vi "RFmx_An_ACP_Disp.vi"(6 "ACP_Values":dbl[](array[numeric]) format="%#_6p", 8 "Int_Bandwidth":dbl[](array[numeric]) format="%#_6p", 9 "Offsets":dbl[](array[numeric]) format="%#_6p", 10 "SignalBandwidth":dbl format="%#_6p", 11 "Input_Waveform":cluster{"x0":dbl, "dx":dbl, "y":sgl[]}) -> (3 "Waveform Graph 2":cluster{"x0":dbl, "dx":dbl, "y":sgl[]}[](graph))   [LabVIEW 2014]
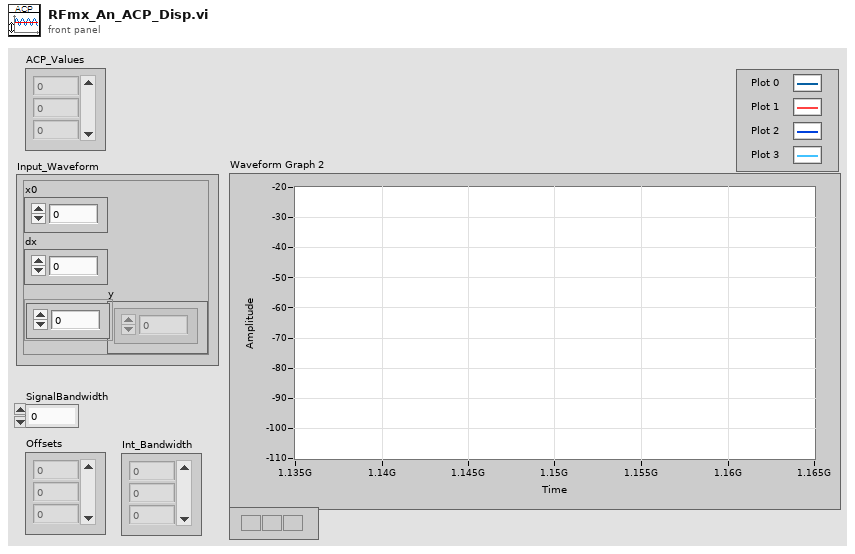
[diagram p1: front panel]
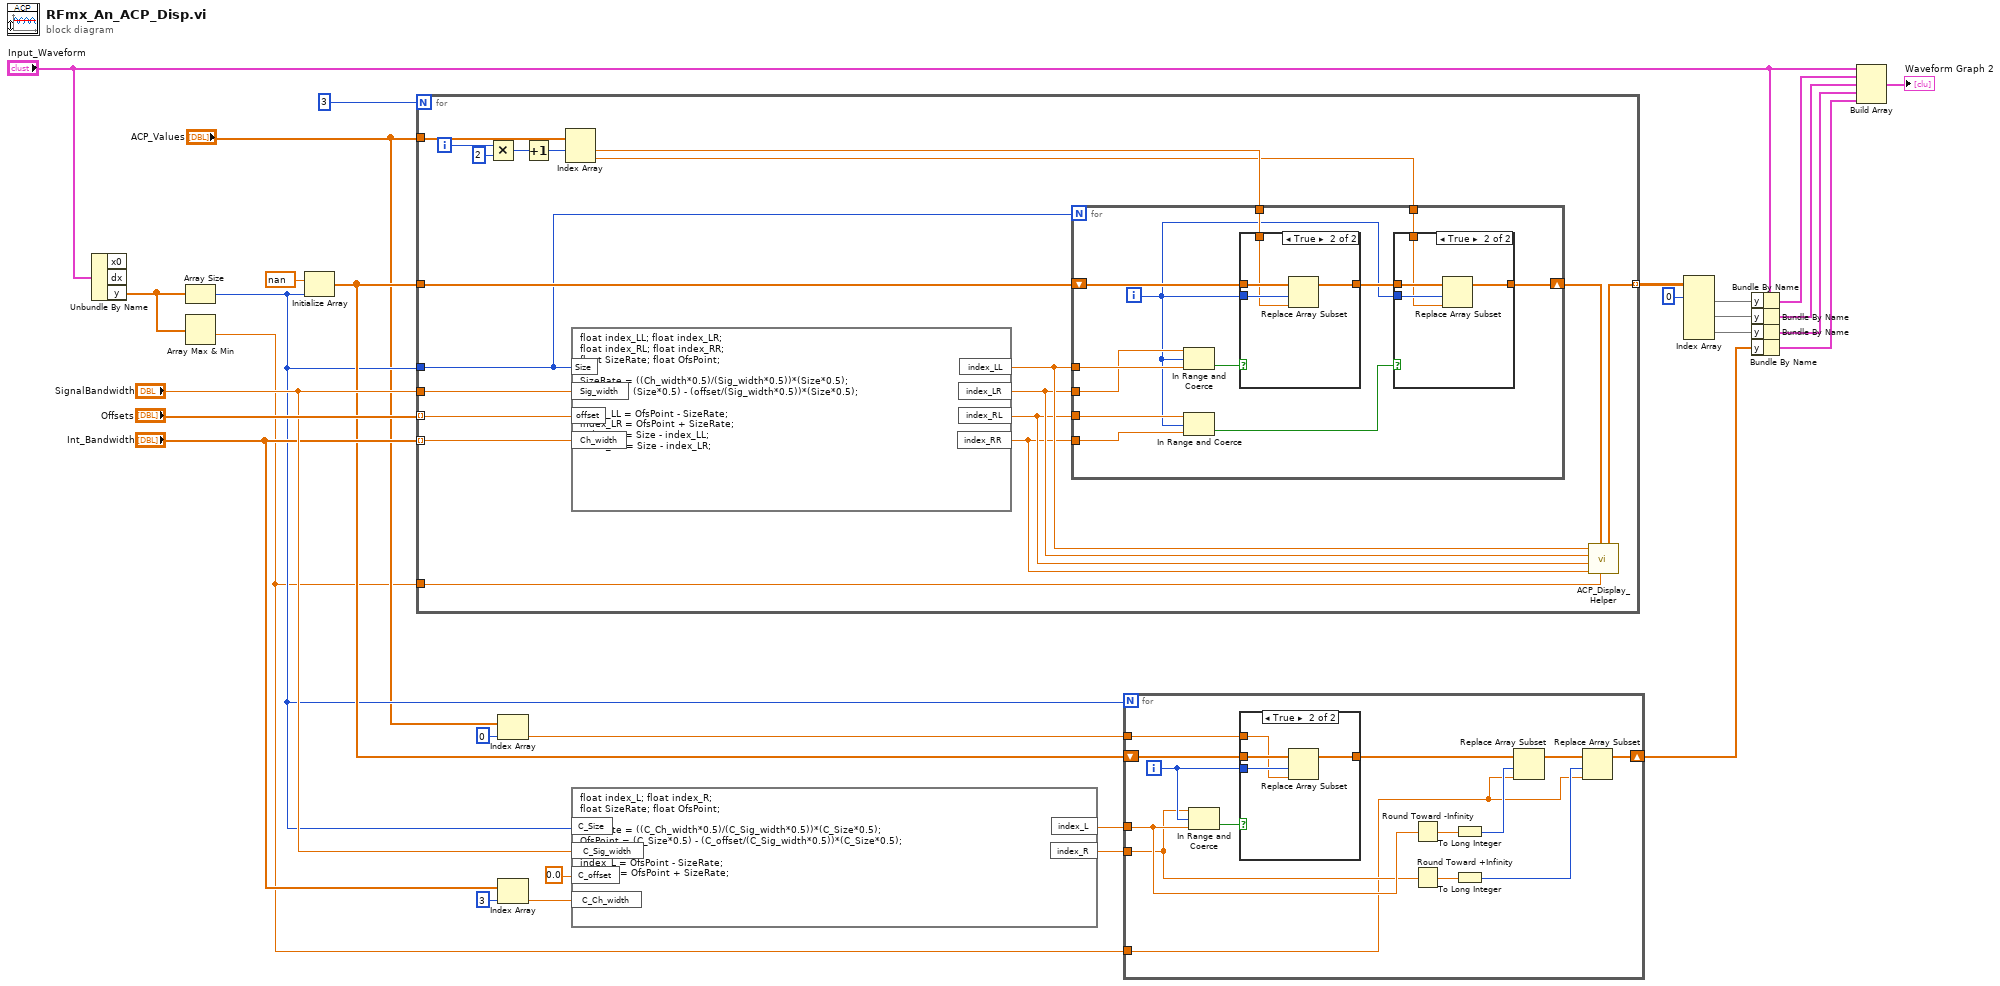
[diagram p0: block diagram]
diagram:
  n1 = Unbundle By Name("Input_Waveform") -> ("y"=w18:sgl[])  [unwired: 2 out]
  n2 = Array Size(array=w18) -> (size(s)=w8:i32)
  n3 = Array Max & Min(array=w18) -> (min value=w3:sgl)  [unwired: 3 out]
  n4 = Initialize Array(nan ("element"), w8) -> (w9:dbl[])
  n5 = for {
    N: 3 -> [_]
    tunnel: "SignalBandwidth" -> [w48]
    tunnel: "Offsets" -> [w47] mode=indexing
    tunnel: "Int_Bandwidth" -> [w46] mode=indexing
    tunnel: [w43] -> w26 mode=indexing
    tunnel: w9 -> [w45]
    tunnel: "ACP_Values" -> [w40]
    tunnel: w8 -> [w44]
    tunnel: w3 -> [w41]
    i -> [w33]
    n6 = Multiply(x=w33, y=2) -> (x*y=w38:i32)
    n7 = Increment(x=w38) -> (x+1=w30:i32)
    n8 = Index Array(array=w40, index #1=w30) -> (element #1=w32:dbl, element #2=w31:dbl)  [unwired: 1 in]
    n9 = formula code="float index_LL; float index_LR;\nfloat index_RL; float index_RR; \nfloat SizeRate; float OfsPoint;\n\nSizeRate = ((Ch_width*0.5)/(Sig_width*0.5))*(Size*0.5);\nOfsPoint = (Size*0.5) - (offset/(Sig_width*0.5))*(Size*0.5);\n\nindex_LL = OfsPoint - SizeRate;\nindex_LR = OfsPoint + SizeRate;\nindex_RL = Size - index_LL;\nindex_RR = Size - index_LR;"("Sig_width"=w48, "offset"=w47, "Ch_width"=w46, "Size"=w44) -> ("index_LL"=w37:dbl, "index_LR"=w36:dbl, "index_RL"=w35:dbl, "index_RR"=w34:dbl)
    n10 = for {
      N: w44 -> [_]
      shift-right: [w50] -> w42
      shift-left: w45 -> [w59]
      tunnel: w37 -> [w60]
      tunnel: w35 -> [w57]
      tunnel: w34 -> [w58]
      tunnel: w36 -> [w56]
      tunnel: w32 -> [w55]
      tunnel: w31 -> [w49]
      i -> [w51]
      n11 = In Range and Coerce(upper limit=w56, x=w51, lower limit=w60) -> (In Range?=w54:bool)  [unwired: 1 out]
      n12 = In Range and Coerce(upper limit=w57, x=w51, lower limit=w58) -> (In Range?=w52:bool)  [unwired: 1 out]
      n13 = case shown="True" w54 {
        tunnel: w59 -> [w66 w70]
        tunnel: w51 -> [_ w69]
        tunnel: [w66 w68] -> w53
        tunnel: w55 -> [_ w67]
        frame False {
        }
        frame True {
          n14 = Replace Array Subset(array=w70, new element=w67, index=w69) -> (w68:dbl[])
        }
      }
      n15 = case shown="True" w52 {
        tunnel: w53 -> [w61 w65]
        tunnel: w51 -> [_ w64]
        tunnel: [w61 w63] -> w50
        tunnel: w49 -> [_ w62]
        frame False {
        }
        frame True {
          n16 = Replace Array Subset(array=w65, new element=w62, index=w64) -> (w63:dbl[])
        }
      }
    }
    n17 = call "ACP_Display_Helper.vi"("Min"=w41, "Mask"=w42, "RR"=w34, "RL"=w35, "LR"=w36, "LL"=w37) -> ("Mask_Out"=w43:dbl[])  [unwired: 5 in]
  }
  n18 = Index Array(array="ACP_Values", index=0) -> (element=w2:dbl)
  n19 = Index Array(array="Int_Bandwidth", index=3) -> (element=w12:dbl)
  n20 = formula code="float index_L; float index_R;\nfloat SizeRate; float OfsPoint;\n\nSizeRate = ((C_Ch_width*0.5)/(C_Sig_width*0.5))*(C_Size*0.5);\nOfsPoint = (C_Size*0.5) - (C_offset/(C_Sig_width*0.5))*(C_Size*0.5);\n\nindex_L = OfsPoint - SizeRate;\nindex_R = OfsPoint + SizeRate;"("C_Sig_width"="SignalBandwidth", "C_offset"=0.0 ("input variable"), "C_Ch_width"=w12, "C_Size"=w8) -> ("index_L"=w6:dbl, "index_R"=w7:dbl)
  n21 = for {
    N: w8 -> [_]
    shift-right: [w72] -> w1
    shift-left: w9 -> [w84]
    tunnel: w7 -> [w74]
    tunnel: w6 -> [w75]
    tunnel: w3 -> [w73]
    tunnel: w2 -> [w71]
    i -> [w82]
    n22 = In Range and Coerce(upper limit=w74, x=w82, lower limit=w75) -> (In Range?=w83:bool)  [unwired: 1 out]
    n23 = case shown="True" w83 {
      tunnel: w84 -> [w85 w89]
      tunnel: w82 -> [_ w88]
      tunnel: [w85 w87] -> w76
      tunnel: w71 -> [_ w86]
      frame False {
      }
      frame True {
        n24 = Replace Array Subset(array=w89, new element=w86, index=w88) -> (w87:dbl[])
      }
    }
    n25 = Round Toward -Infinity(1:w75) -> (0:w81:dbl)
    n26 = Round Toward +Infinity(x=w74) -> (ceil(x): smallest int >= x=w80:dbl)
    n27 = To Long Integer(number=w81) -> (32bit integer=w79:i32)
    n28 = To Long Integer(number=w80) -> (32bit integer=w77:i32)
    n29 = Replace Array Subset(array=w76, new element=w73, index=w79) -> (w78:dbl[])
    n30 = Replace Array Subset(array=w78, new element=w73, index=w77) -> (w72:dbl[])
  }
  n31 = Index Array(array=w26, index (row) #1=0 ("index (row)")) -> (element #1=w23:dbl[], element #2=w22:dbl[], element #3=w21:dbl[])  [unwired: 5 in]
  n32 = Bundle By Name(cluster="Input_Waveform", "y"=w23) -> (w24:cluster{"x0":dbl, "dx":dbl, "y":sgl[]})
  n33 = Bundle By Name(cluster="Input_Waveform", "y"=w22) -> (w20:cluster{"x0":dbl, "dx":dbl, "y":sgl[]})
  n34 = Bundle By Name(cluster="Input_Waveform", "y"=w21) -> (w19:cluster{"x0":dbl, "dx":dbl, "y":sgl[]})
  n35 = Bundle By Name(cluster="Input_Waveform", "y"=w1) -> (w17:cluster{"x0":dbl, "dx":dbl, "y":sgl[]})
  n36 = Build Array("Input_Waveform", w24, w20, w19, w17) -> (→"Waveform Graph 2":cluster{"x0":dbl, "dx":dbl, "y":sgl[]}[])
